vi "manual alum dose.vi"(5 "Time":dbl format="%.2f", 6 "sensor value":dbl, 7 "Set Points":dbl[](array[numeric])) -> (3 "fraction on":dbl)   [LabVIEW 2010]
panel:
  out "output cluster":T1
  in  "tubing size":enum16{"13", "14", "16", "25", "17", "18"}(ring)
  in  "Pump":T1 {"flow rate" format="%.2f"}
  # "plant flow (mL/min)\nalum stock concentration (mg/L)\nalum dose (mg/L)\ntubing size"
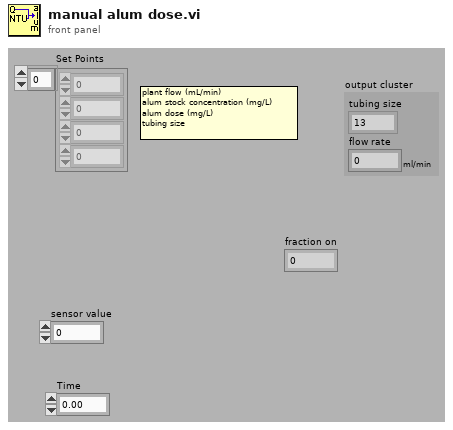
[diagram p1: front panel]
types:
  T1 = cluster{"tubing size":enum16{"13", "14", "16", "25", "17", "18"}, "flow rate":dbl[unit]}
  T2 = cluster{"Set Points[0]":dbl, "Set Points[1]":dbl, "Set Points[2]":dbl, "Set Points[3]":dbl}
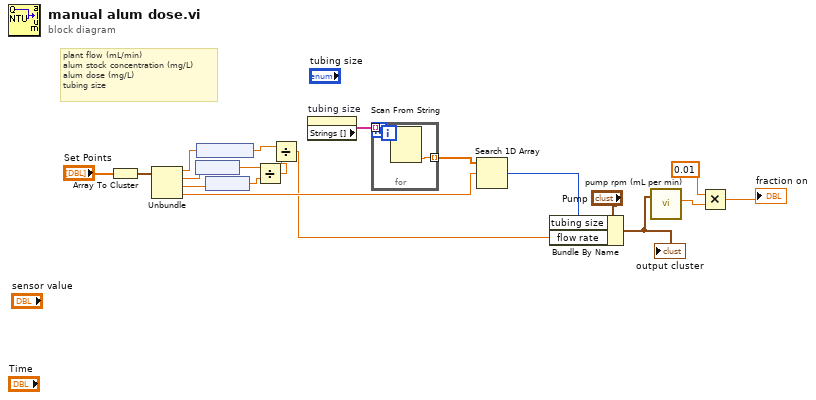
[diagram p0: block diagram]
diagram:
  # "plant flow (mL/min)\nalum stock concentration (mg/L)\nalum dose (mg/L)\ntubing size"
  n1 = Array To Cluster(array="Set Points") -> (cluster=w18:T2)
  n2 = Unbundle(w18) -> ("Set Points[0]"=w8:dbl, "Set Points[1]"=w7:dbl, "Set Points[2]"=w6:dbl, "Set Points[3]"=w16:dbl)
  n3 = node(w7) -> (w4:dbl[unit])
  n4 = node(w8) -> (w3:dbl[unit])
  n5 = node(w6) -> (w5:dbl[unit])
  n6 = Divide(x=w4, y=w5) -> (x/y=w2:dbl)
  n7 = Divide(x=w3, y=w2) -> (x/y=w1:dbl[unit])
  n8 = property on="tubing size" class="Enum (strict)"() -> ("Strings []"=w17:string[])  [unwired: 2 in, 2 out]
  n9 = for {
    tunnel: w17 -> [w21] mode=indexing
    tunnel: [w20] -> w15 mode=indexing
    n10 = Scan From String(input string=w21) -> (output 1=w20:dbl)  [unwired: 4 in, 3 out]
  }
  n11 = Search 1D Array(1D array=w15, element=w16) -> (index of element=w12:i32)  [unwired: 1 in]
  n12 = Bundle By Name(cluster="Pump", "tubing size"=w12, "flow rate"=w1) -> (w13:T1)
  "output cluster" <- w13
  n13 = call "pump rpm (mL per min).vi"("Pump"=w13) -> ("pump speed (rpm)"=w11:dbl)  [unwired: 1 in, 3 out]
  n14 = Multiply(x=0.01, y=w11) -> (x*y=→"fraction on":dbl)
